vi "Answer Request.vi"(7 "Data":variant, 8 "error in (no error)":errorcluster, 9 "Function ID":u8, 10 "Stack ID":u8, 11 "IP Connection in":refnum<class "IP Connection.lvclass">) -> (0 "error out":errorcluster, 3 "IP Connection out":refnum<class "IP Connection.lvclass">)   [LabVIEW 2011, in "Tinkerforge.lvlib" / "IP Connection.lvclass"]
doc: "This VI answeres a former request if still pending."
uses:
  IP Connection.lvclass
  IP Connection.lvclass/IP Connection.ctl
  Type Definitions/Request Type.ctl
  Type Definitions/Answer.ctl
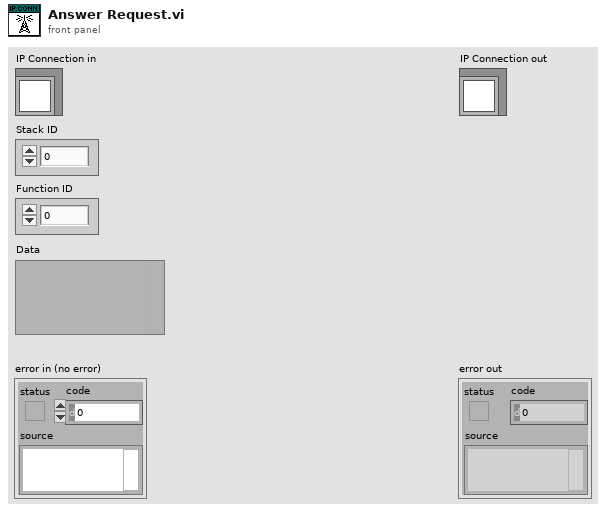
[diagram p1: front panel]
types:
  T1 = typedef "Tinkerforge.lvlib/IP Connection.lvclass/Request Type.ctl" = enum8{"Invalid", "Write"}
  T2 = typedef "Tinkerforge.lvlib/IP Connection.lvclass/Answer.ctl" = cluster{"Request GUID":string, "Request Type":T1, "Sucessful":bool, "Data":variant, "Error":errorcluster}
  T3 = typedef "Tinkerforge.lvlib/IP Connection.lvclass/Request Identifier.ctl" = cluster{"Stack ID":u8, "Function ID":u8, "Request GUID":string, "Remaining Timeout":i32}
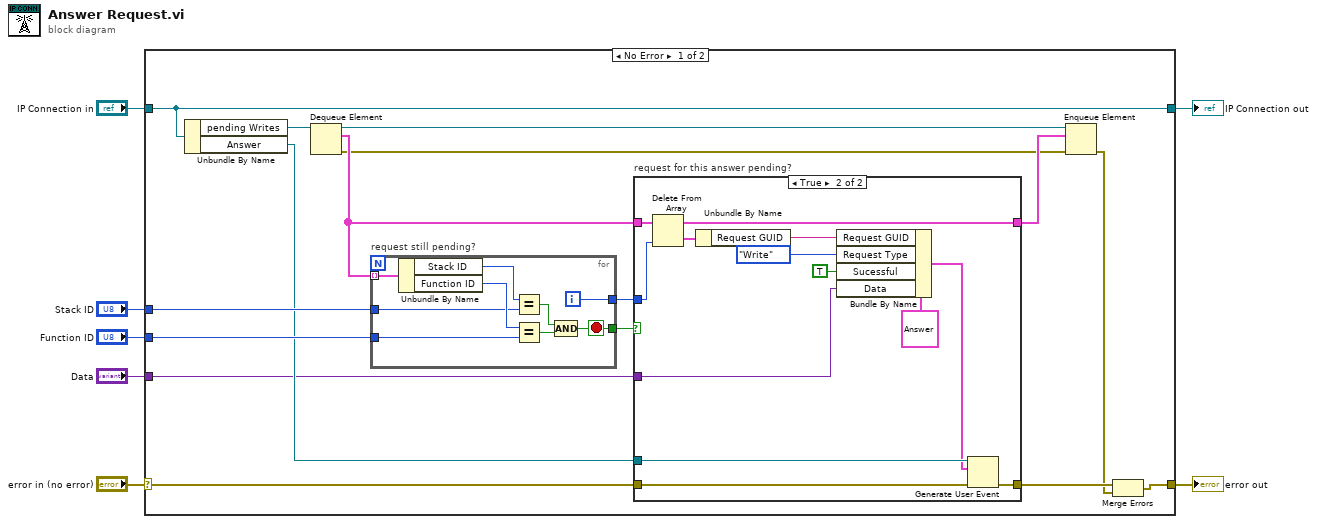
[diagram p0: block diagram]
diagram:
  n1 = case shown="No Error" "error in (no error)" {
    selector: "error in (no error)" -> [w13 w49]
    tunnel: [w8 w49] -> w6
    tunnel: [w23 w48] -> w4
    tunnel: "IP Connection in" -> [w23 w48]
    tunnel: "Stack ID" -> [w21 _]
    tunnel: "Function ID" -> [w20 _]
    tunnel: "Data" -> [w11 _]
    frame No Error {
      n2 = Unbundle By Name(w23) -> ("pending Writes"=w22:refnum<queue>, "Answer"=w12:refnum<user-event>)
      n3 = Dequeue Element(queue=w22) -> (queue out=w16:refnum<queue>, element=w19:T3[], error out=w14:errorcluster)  [unwired: 2 in, 1 out]
      n4 = for "request still pending?" {
        tunnel: w19 -> [w47] mode=indexing
        tunnel: w21 -> [w44]
        tunnel: w20 -> [w43]
        tunnel: [w40] -> w17
        tunnel: [w39] -> w18
        i -> [w40]
        stop <- w39 stop-if-true
        n5 = Unbundle By Name(w47) -> ("Stack ID"=w46:u8, "Function ID"=w45:u8)
        n6 = Equal?(x=w46, y=w44) -> (x = y?=w42:bool)
        n7 = Equal?(x=w45, y=w43) -> (x = y?=w41:bool)
        n8 = Compound Arithmetic op=AND(w42, w41) -> (w39:bool)
      }
      n9 = case "request for this answer pending?" shown="True" w18 {
        tunnel: w19 -> [w25 w38]
        tunnel: w17 -> [_ w37]
        tunnel: [w25 w36] -> w15
        tunnel: w13 -> [w24 w28]
        tunnel: w12 -> [_ w34]
        tunnel: w11 -> [_ w29]
        tunnel: [w24 w26] -> w10
        frame False {
        }
        frame True {
          n10 = Delete From Array(array=w38, index=w37) -> (deleted portion=w35:T3, array with subset deleted=w36:T3[])  [unwired: 1 in]
          n11 = Unbundle By Name(w35) -> ("Request GUID"=w32:string)
          n12 = Bundle By Name(cluster=T2 {"Request GUID"="", "Request Type"=enum."Invalid", "Sucessful"=FALSE, "Data"=variant, "Error"={"status"=FALSE, "code"=0, "source"=""}} ("event data"), "Request GUID"=w32, "Request Type"=Request_Type."Write", "Sucessful"=TRUE, "Data"=w29) -> (w27:T2)
          n13 = Generate User Event(user event=w34, event data cluster=w27, error in=w28) -> (error out=w26:errorcluster)  [unwired: 1 out]
        }
      }
      n14 = Enqueue Element(queue=w16, element=w15, error in (no error)=w14) -> (error out=w9:errorcluster)  [unwired: 1 in, 2 out]
      n15 = Merge Errors(w10, w9) -> (w8:errorcluster)
    }
    frame Error {
    }
  }
  "error out" <- w6
  "IP Connection out" <- w4
